vi "CheckForBibDuplicate.vi"(10 "ArrayOfDuplicateBibNumbers":string[](array[string]), 11 "ArrayOfBibs":string[](array[string])) -> (3 "ArrayOfDuplicateBibNumbers":string[](array[string]))   [LabVIEW 2020]
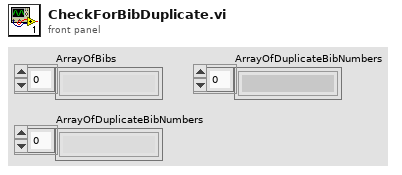
[diagram p1: front panel]
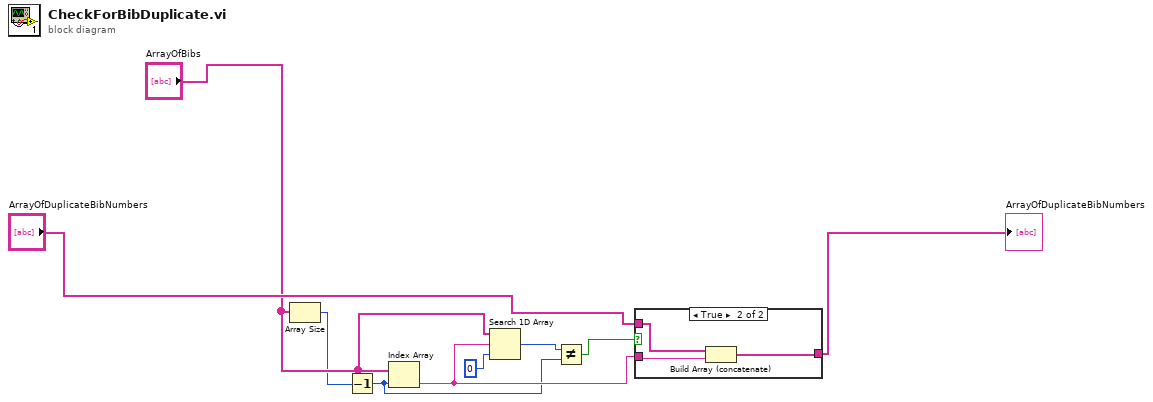
[diagram p0: block diagram]
diagram:
  n1 = Array Size(array="ArrayOfBibs") -> (size(s)=w1:i32)
  n2 = Decrement(x=w1) -> (x-1=w5:i32)
  n3 = Index Array(array="ArrayOfBibs", index=w5) -> (element=w7:string)
  n4 = Search 1D Array(1D array="ArrayOfBibs", element=w7, start index (0)=0) -> (index of element=w4:i32)
  n5 = Not Equal?(x=w4, y=w5) -> (x != y?=w6:bool)
  n6 = case shown="True" w6 {
    tunnel: w7 -> [_ w12]
    tunnel: "ArrayOfDuplicateBibNumbers" -> [w10 w13]
    tunnel: [w10 w11] -> w8
    frame False {
    }
    frame True {
      n7 = Build Array (concatenate)(w13, w12) -> (w11:string[])
    }
  }
  "ArrayOfDuplicateBibNumbers" <- w8
